vi "Set VI Printing Options.vi"(6 "margins":T4={"override VI margins (false)"=FALSE, "margins (1.00)"={"top"=1.0, "left"=1.0, "right"=1.0, "bottom"=1.0}, "measurement system (default)"=0} {"measurement system (default)" items=["Default", "US", "Metric"]; "margins (1.00)"."right" format="%.2f"; "margins (1.00)"."bottom" format="%.2f"; "margins (1.00)"."top" format="%.2f"; "margins (1.00)"."left" format="%.2f"}, 7 "page header options":T1={"page headers (unchanged)"=0, "page header content options"={"Include VI Name"=TRUE, "Include VI Path"=TRUE, "Include Last Modification Date"=TRUE, "Include Date Printed"=TRUE, "Include Page Number"=TRUE, "Include VI Icon"=TRUE}} {"page headers (unchanged)" items=["Unchanged", "Include page headers", "Do not include page headers"]}, 8 "error in (no error)":errorcluster, 9 "orientation (unchanged)":T7 items=["Unchanged", "portrait", "landscape"], 10 "panel scaling for page (unchanged)":T8 items=["Unchanged", "No Scaling", "Scale front panel to fit"], 11 "VI Refnum":refnum<vi>) -> (0 "error out":errorcluster, 3 "VI Refnum out":refnum<vi>)   [LabVIEW 2017, in "NI_ReportGenerationCore.lvlib"]
uses:
  <vilib>/Utility/NIReport.llb/NI_ReportGenerationCore.lvlib
  <vilib>/printing/EasyPrintingControls.llb/panel_scaling_for_page.ctl
  <vilib>/printing/EasyPrintingControls.llb/orientation.ctl
  <vilib>/printing/EasyPrintingControls.llb/margins.ctl
  <vilib>/printing/EasyPrintingControls.llb/margin_values.ctl
  <vilib>/printing/EasyPrintingControls.llb/measurement_system.ctl
  <vilib>/printing/EasyPrintingControls.llb/page_header_options.ctl
  <vilib>/printing/EasyPrintingControls.llb/page_headers.ctl
  <vilib>/printing/EasyPrintingControls.llb/page_header_content_options.ctl
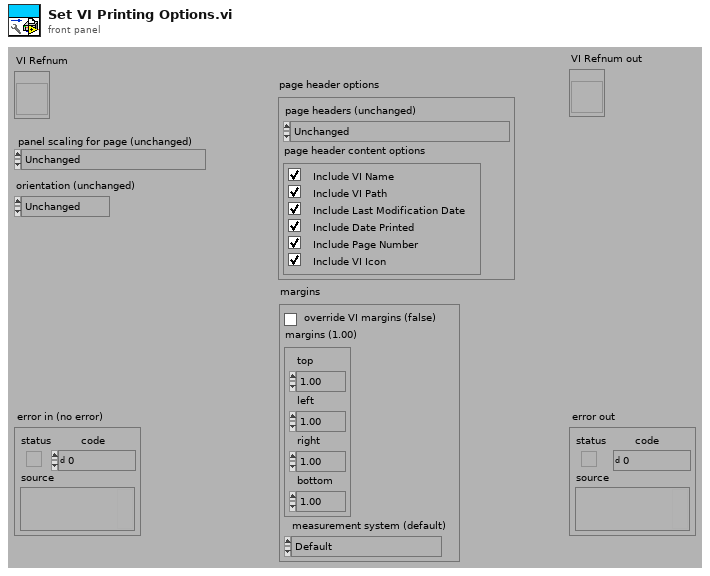
[diagram p1: front panel]
types:
  T1 = typedef "NI_ReportGenerationCore.lvlib/page_header_options.ctl" = cluster{"page headers (unchanged)":T2, "page header content options":T3}
  T2 = typedef "NI_ReportGenerationCore.lvlib/page_headers.ctl" = u16
  T3 = typedef "NI_ReportGenerationCore.lvlib/page_header_content_options.ctl" = cluster{"Include VI Name":bool, "Include VI Path":bool, "Include Last Modification Date":bool, "Include Date Printed":bool, "Include Page Number":bool, "Include VI Icon":bool}
  T4 = typedef "NI_ReportGenerationCore.lvlib/margins.ctl" = cluster{"override VI margins (false)":bool, "margins (1.00)":T5, "measurement system (default)":T6}
  T5 = typedef "NI_ReportGenerationCore.lvlib/margin_values.ctl" = cluster{"top":dbl, "left":dbl, "right":dbl, "bottom":dbl}
  T6 = typedef "NI_ReportGenerationCore.lvlib/measurement_system.ctl" = u16
  T7 = typedef "NI_ReportGenerationCore.lvlib/orientation.ctl" = u16
  T8 = typedef "NI_ReportGenerationCore.lvlib/panel_scaling_for_page.ctl" = u16
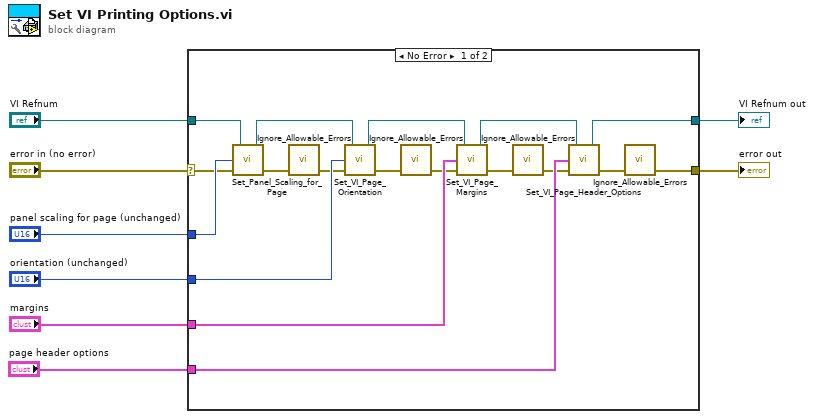
[diagram p0: block diagram]
diagram:
  n1 = case shown="No Error" "error in (no error)" {
    selector: "error in (no error)" -> [w25 w28]
    tunnel: [w14 w28] -> w7
    tunnel: [w9 w27] -> w5
    tunnel: "VI Refnum" -> [w13 w27]
    tunnel: "panel scaling for page (unchanged)" -> [w26 _]
    tunnel: "orientation (unchanged)" -> [w24 _]
    tunnel: "margins" -> [w23 _]
    tunnel: "page header options" -> [w22 _]
    frame No Error {
      n2 = call <vilib>:"Set_Panel_Scaling_for_Page.vi"("error in"=w25, "panel scaling for page (unchanged)"=w26, "VI Refnum"=w13) -> ("error out"=w21:errorcluster, "VI Refnum out"=w12:refnum<vi>)
      n3 = call <vilib>:"Ignore_Allowable_Errors.vi"("error in (no error)"=w21) -> ("error out"=w20:errorcluster)  [unwired: 10 in]
      n4 = call <vilib>:"Set_VI_Page_Orientation.vi"("error in"=w20, "orientation (unchanged)"=w24, "VI Refnum"=w12) -> ("error out"=w19:errorcluster, "VI Refnum out"=w11:refnum<vi>)
      n5 = call <vilib>:"Ignore_Allowable_Errors.vi"("error in (no error)"=w19) -> ("error out"=w18:errorcluster)  [unwired: 10 in]
      n6 = call <vilib>:"Set_VI_Page_Margins.vi"("error in (no error)"=w18, "margins"=w23, "VI Refnum"=w11) -> ("error out"=w17:errorcluster, "VI Refnum out"=w10:refnum<vi>)
      n7 = call <vilib>:"Ignore_Allowable_Errors.vi"("error in (no error)"=w17) -> ("error out"=w16:errorcluster)  [unwired: 10 in]
      n8 = call <vilib>:"Set_VI_Page_Header_Options.vi"("error in"=w16, "page header options"=w22, "VI Refnum"=w10) -> ("error out"=w15:errorcluster, "VI Refnum out"=w9:refnum<vi>)
      n9 = call <vilib>:"Ignore_Allowable_Errors.vi"("error in (no error)"=w15) -> ("error out"=w14:errorcluster)  [unwired: 10 in]
    }
    frame Error {
    }
  }
  "error out" <- w7
  "VI Refnum out" <- w5
